vi "测棒价值数据处理.vi"() -> ()   [LabVIEW 2020]
uses:
  <vilib>/Utility/miscctls.llb/LVAnnotationListTypeDef.ctl
  <vilib>/Utility/miscctls.llb/LVRowAndColumnTypeDef.ctl
  <vilib>/Utility/inputDevices.llb/mouseAcquire.vi
  <vilib>/Analysis/NI_AALPro.lvlib
panel:
  out "准临界周期 (s)":dbl[](array[numeric])
  out "拟合反应性 (pcm)":dbl[](array[numeric])
  out "终端反应性 (pcm)":dbl[](array[numeric])
  out "实时反应性 (pcm)":dbl[](array[numeric])
  in  "刻棒选择":u16(ring)
  in  "棒位偏移":dbl(slide) min=-0.1 max=0.1 step=0.001 scale=-0.1..0.1 scale format="%#.3g"
  in  "反应性标尺":bool
  in  "Min+":bool
  in  "Min-":bool
  in  "Max+":bool
  in  "Max-":bool
  out "历史波形图":dbl[][](graph)
  in  "曲线标尺":bool[](array[boolean])=[TRUE, TRUE]
  in  "曲线隐显":bool[](array[boolean])=[TRUE, TRUE, FALSE, FALSE, FALSE]
  out "终端":i32
  out "动态段":i32
  out "左选标时刻":timestamp
  out "总时长":dbl
  in  "开始计算":bool
  in  "重选文件":bool
  in  "退出程序":bool
  out "filepath":path caption="数据文件路径和名称"
  out "数据采集起止时间":string
  out "临界段":i32
  out "稳定临界":i32
  out "开始落棒":i32
  out "Table":string[][](table) caption="总价值汇总"
  in  "保存表格":bool
  in  "添加记录":bool
  in  "选项卡控件":enum32{"动态段数据", "动态段曲线"}(tab)
  out "ValueTable":string[][](table)=[["102.000000", "NaN", "-348.352776", "7.241968"], ["101.000000", "NaN", "2474.422828", "-4.851056"], ["100.000000", "NaN", "-622.831158", "13.483680"], ["99.000000", "NaN", "-527.371545", "-19.758989"], ["98.000000", "NaN", "-567.571450", "-10.039112"], ["97.000000", "NaN", "-587.204400", "6.175295"], ["96.000000", "NaN", "-348.236291", "13.619997"], ["95.000000", "NaN", "2458.347144", "-10.205061"], ["94.000000", "NaN", "-622.921258", "5.615908"], ["93.000000", "NaN", "-527.356225", "2.660273"], ["92.000000", "NaN", "-567.556832", "-0.988388"], ["91.000000", "NaN", "-587.208474", "-1.085916"], ["90.000000", "NaN", "-351.120934", "-4.397986"], ["89.000000", "NaN", "2304.904029", "2.228443"], ["88.000000", "NaN", "-618.140019", "-11.538202"], ["87.000000", "NaN", "-525.138329", "-21.395784"], ["86.000000", "NaN", "-565.982171", "-3.062838"], ["85.000000", "NaN", "-585.993836", "-11.582806"], ["84.000000", "NaN", "-356.379876", "-4.609295"], ["83.000000", "NaN", "2014.719947", "-24.758602"], ["82.000000", "NaN", "-607.663750", "-9.042081"], ["81.000000", "NaN", "-519.521004", "-11.768277"], ["80.000000", "NaN", "-561.868691", "-21.104680"], ["79.000000", "NaN", "-582.802468", "-20.175712"], ["78.000000", "NaN", "-370.631005", "-22.793518"], ["77.000000", "NaN", "1553.766334", "-35.673673"], ["76.000000", "NaN", "-582.848588", "-30.558160"], ["75.000000", "NaN", "-506.097573", "-43.964250"], ["74.000000", "NaN", "-552.008980", "-40.812654"], ["73.000000", "NaN", "-575.099190", "-48.470411"], ["72.000000", "NaN", "-396.508813", "-49.474470"], ["71.000000", "NaN", "1094.646827", "-51.345674"], ["70.000000", "NaN", "-538.590142", "-76.883382"], ["69.000000", "NaN", "-482.233040", "-72.882963"], ["68.000000", "NaN", "-534.351227", "-82.754262"], ["67.000000", "NaN", "-561.206460", "-96.003896"], ["66.000000", "NaN", "-437.894280", "-90.676832"], ["65.000000", "NaN", "754.871925", "-96.218252"], ["64.000000", "NaN", "-475.456872", "-112.709539"], ["63.000000", "NaN", "-448.215874", "-123.690824"], ["62.000000", "NaN", "-508.844033", "-113.615911"], ["61.000000", "NaN", "-540.932023", "-115.695623"], ["60.000000", "NaN", "-505.853066", "-123.674741"], ["59.000000", "NaN", "533.852882", "-168.205152"], ["58.000000", "NaN", "-398.363793", "-171.710203"], ["57.000000", "NaN", "-411.278634", "-156.485715"], ["56.000000", "NaN", "-503.550530", "-189.779630"], ["55.000000", "NaN", "-558.146439", "-200.472120"], ["54.000000", "NaN", "-602.408646", "-192.425687"], ["53.000000", "NaN", "-639.806430", "-193.738553"], ["52.000000", "NaN", "-674.476414", "-191.523603"], ["51.000000", "NaN", "-700.441693", "-249.642133"], ["50.000000", "NaN", "-724.497986", "-241.971433"], ["49.000000", "NaN", "-754.798043", "-266.290555"], ["48.000000", "NaN", "-775.840317", "-264.434385"], ["47.000000", "NaN", "-798.536919", "-291.856107"], ["46.000000", "NaN", "-818.504510", "-287.589536"], ["45.000000", "NaN", "-838.204919", "-305.410093"], ["44.000000", "NaN", "-860.447259", "-298.660703"], ["43.000000", "NaN", "-884.024087", "-330.586606"], ["42.000000", "NaN", "-908.885247", "-345.129301"], ["41.000000", "NaN", "-937.339654", "-354.504972"], ["40.000000", "NaN", "-955.449700", "-356.992582"], ["39.000000", "NaN", "-990.566125", "-360.303831"], ["38.000000", "NaN", "-1010.004540", "-374.933347"], ["37.000000", "NaN", "-1043.396813", "-401.850858"], ["36.000000", "NaN", "-1071.659783", "-439.057493"], ["35.000000", "NaN", "-1099.095025", "-406.192869"], ["34.000000", "NaN", "-1152.078759", "-466.934385"], ["33.000000", "NaN", "-1177.829796", "-468.282712"], ["32.000000", "NaN", "-1222.924279", "-456.289701"], ["31.000000", "NaN", "-1264.624718", "-460.500486"], ["30.000000", "NaN", "-1309.989220", "-475.509641"], ["29.000000", "NaN", "-1367.020409", "-503.021970"], ["28.000000", "NaN", "-1422.772057", "-497.549833"], ["27.000000", "NaN", "-1496.451501", "-486.375333"], ["26.000000", "NaN", "-1576.901635", "-506.166898"], ["25.000000", "NaN", "-1667.238000", "-603.034665"], ["24.000000", "NaN", "-1761.502953", "-538.524656"], ["23.000000", "NaN", "-2206.159569", "-566.865903"], ["22.000000", "NaN", "-1641.630273", "-535.883054"], ["21.000000", "NaN", "-1600.580163", "-573.607480"], ["20.000000", "NaN", "-1556.563500", "-559.440488"], ["19.000000", "NaN", "-1515.641564", "-582.165281"], ["18.000000", "NaN", "-1478.138878", "-558.577390"], ["17.000000", "NaN", "-1443.844872", "-665.358335"], ["16.000000", "NaN", "-1412.422997", "-573.492002"], ["15.000000", "NaN", "-1383.463097", "-615.937436"], ["14.000000", "NaN", "-1356.686242", "-644.269102"], ["13.000000", "NaN", "-634.271134", "-622.237424"], ["12.000000", "NaN", "12773.841041", "-573.894834"], ["11.000000", "NaN", "-2338.911156", "-625.372129"], ["10.000000", "NaN", "-1151.127679", "-629.015623"], ["9.000000", "NaN", "-1188.514062", "-614.873228"], ["8.000000", "NaN", "-1188.497399", "-642.504880"], ["7.000000", "NaN", "-1181.560387", "-654.091062"], ["6.000000", "NaN", "-1171.780419", "-630.052976"], ["5.000000", "NaN", "-1160.657616", "-647.022458"], ["4.000000", "NaN", "-1149.016137", "-624.654294"], ["3.000000", "NaN", "-1136.935021", "-613.506833"], ["2.000000", "NaN", "-1124.845116", "-602.012571"], ["1.000000", "NaN", "-777.317902", "-666.974668"]] caption="动态段"
  in  "另存数据":bool
  out "价值曲线":cluster{dbl[], dbl[]}[](graph) caption="（X和Y数组）多曲线"
  out "提示信息":string
  # "手动"
  # "自动"
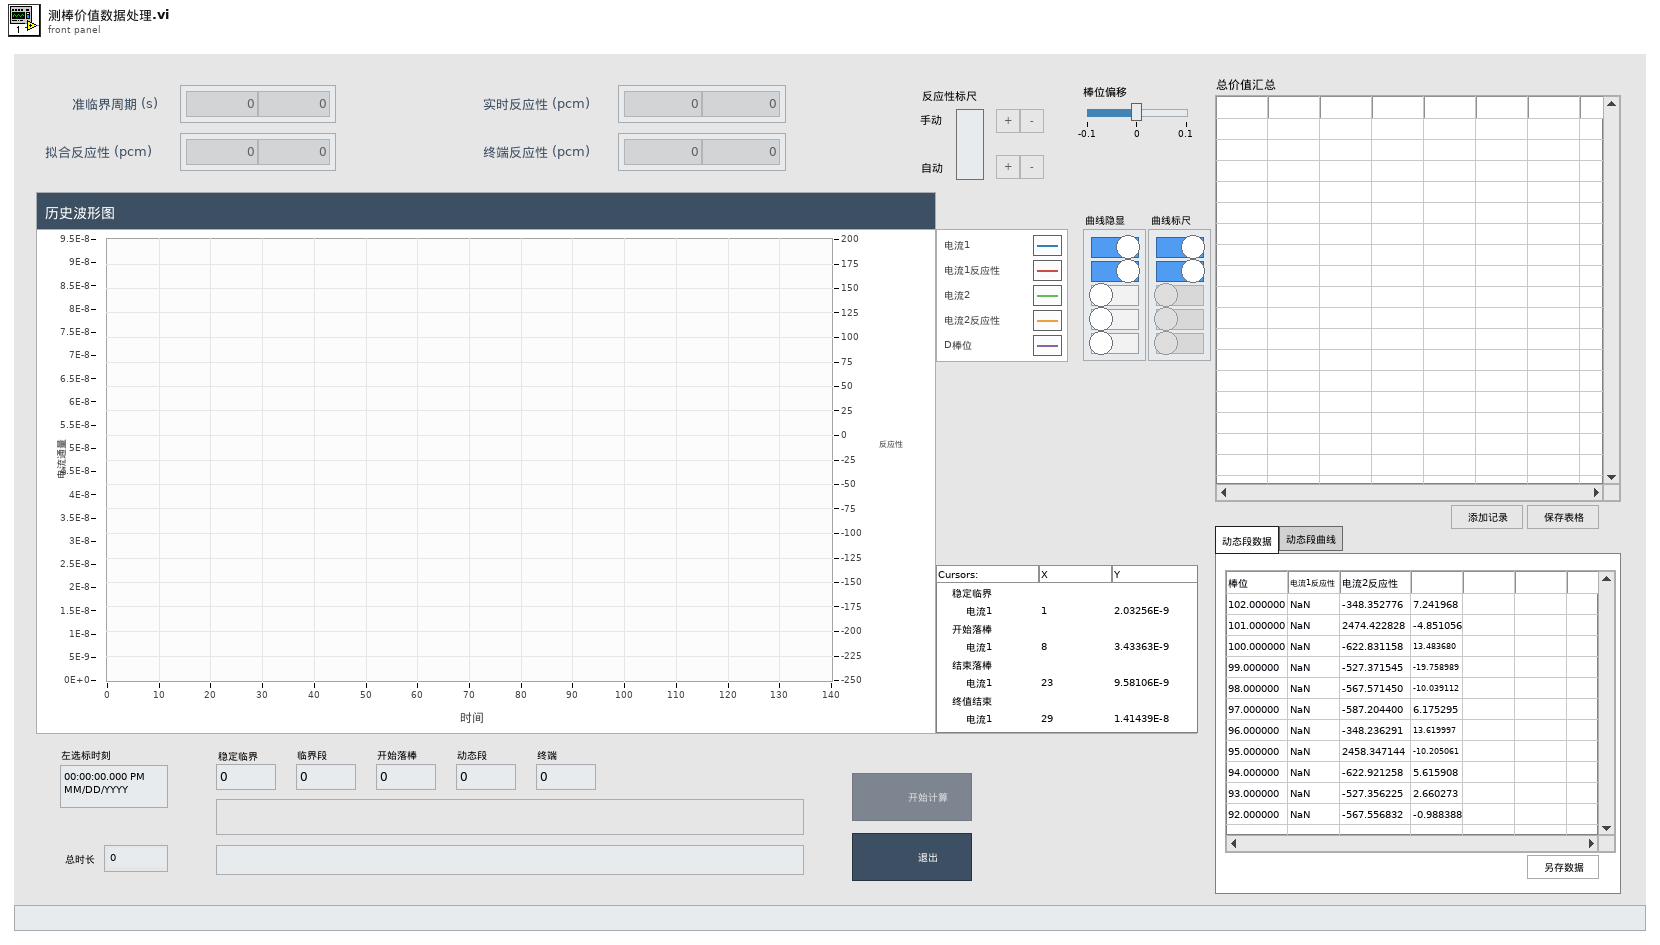
[diagram p1: front panel]
types:
  T1 = enum8{"Enabled", "Disabled", "Disabled and Grayed Out"}
  T2 = typedef "LVAnnotationListTypeDef.ctl" = cluster{"Name":string, "Color":u32, "Style":u8, "Point Style":u8, "Name Visible":bool, "Allow Drag":bool, "Annotation Mode":u32, "Plot":i32, "Index":i32, "Position":cluster{"X":dbl, "Y":dbl}, "X Scale":u32, "Y Scale":u32, "Show Arrow":bool, "Lock Name":bool, "Plot Area":i32, "Label Offset":cluster{"X":dbl, "Y":dbl}}[]
  T3 = cluster{"Name":string, "Color":u32, "Style":u8, "Point Style":u8, "Name Visible":bool, "Allow Drag":bool, "Annotation Mode":u32, "Plot":i32, "Index":i32, "Position":cluster{"X":dbl, "Y":dbl}, "X Scale":u32, "Y Scale":u32, "Show Arrow":bool, "Lock Name":bool, "Plot Area":i32, "Label Offset":cluster{"X":dbl, "Y":dbl}}
  T4 = cluster{"amp min":dbl, "amp max":dbl, "damping min":dbl, "damping max":dbl, "offset min":dbl, "offset max":dbl}
  T5 = enum16{"open", "replace", "create", "open or create", "replace or create", "replace or create with confirmation"}
  T6 = typedef "LVRowAndColumnTypeDef.ctl" = cluster{"Row":i32, "Column":i32}
  T7 = typedef "LVCursorListTypeDef.ctl" = cluster{"Name":string, "Color":u32, "Style":u8, "Point Style":u8, "Name Visible":bool, "Allow Drag":bool, "Cursor Mode":u32, "Plot":i32, "Index":i32, "Position":cluster{"X":dbl, "Y":dbl}, "X Scale":u32, "Y Scale":u32, "Watch Plots":i32[], "Watch All Plots":bool, "Plot Area":i32, "Label Offset":cluster{"X":dbl, "Y":dbl}}[]
  T8 = cluster{"button 1":bool, "button 2":bool, "button 3":bool, "button 4":bool}
  T9 = cluster{"Name":string, "Color":u32, "Style":u8, "Point Style":u8, "Name Visible":bool, "Allow Drag":bool, "Cursor Mode":u32, "Plot":i32, "Index":i32, "Position":cluster{"X":dbl, "Y":dbl}, "X Scale":u32, "Y Scale":u32, "Watch Plots":i32[], "Watch All Plots":bool, "Plot Area":i32, "Label Offset":cluster{"X":dbl, "Y":dbl}}
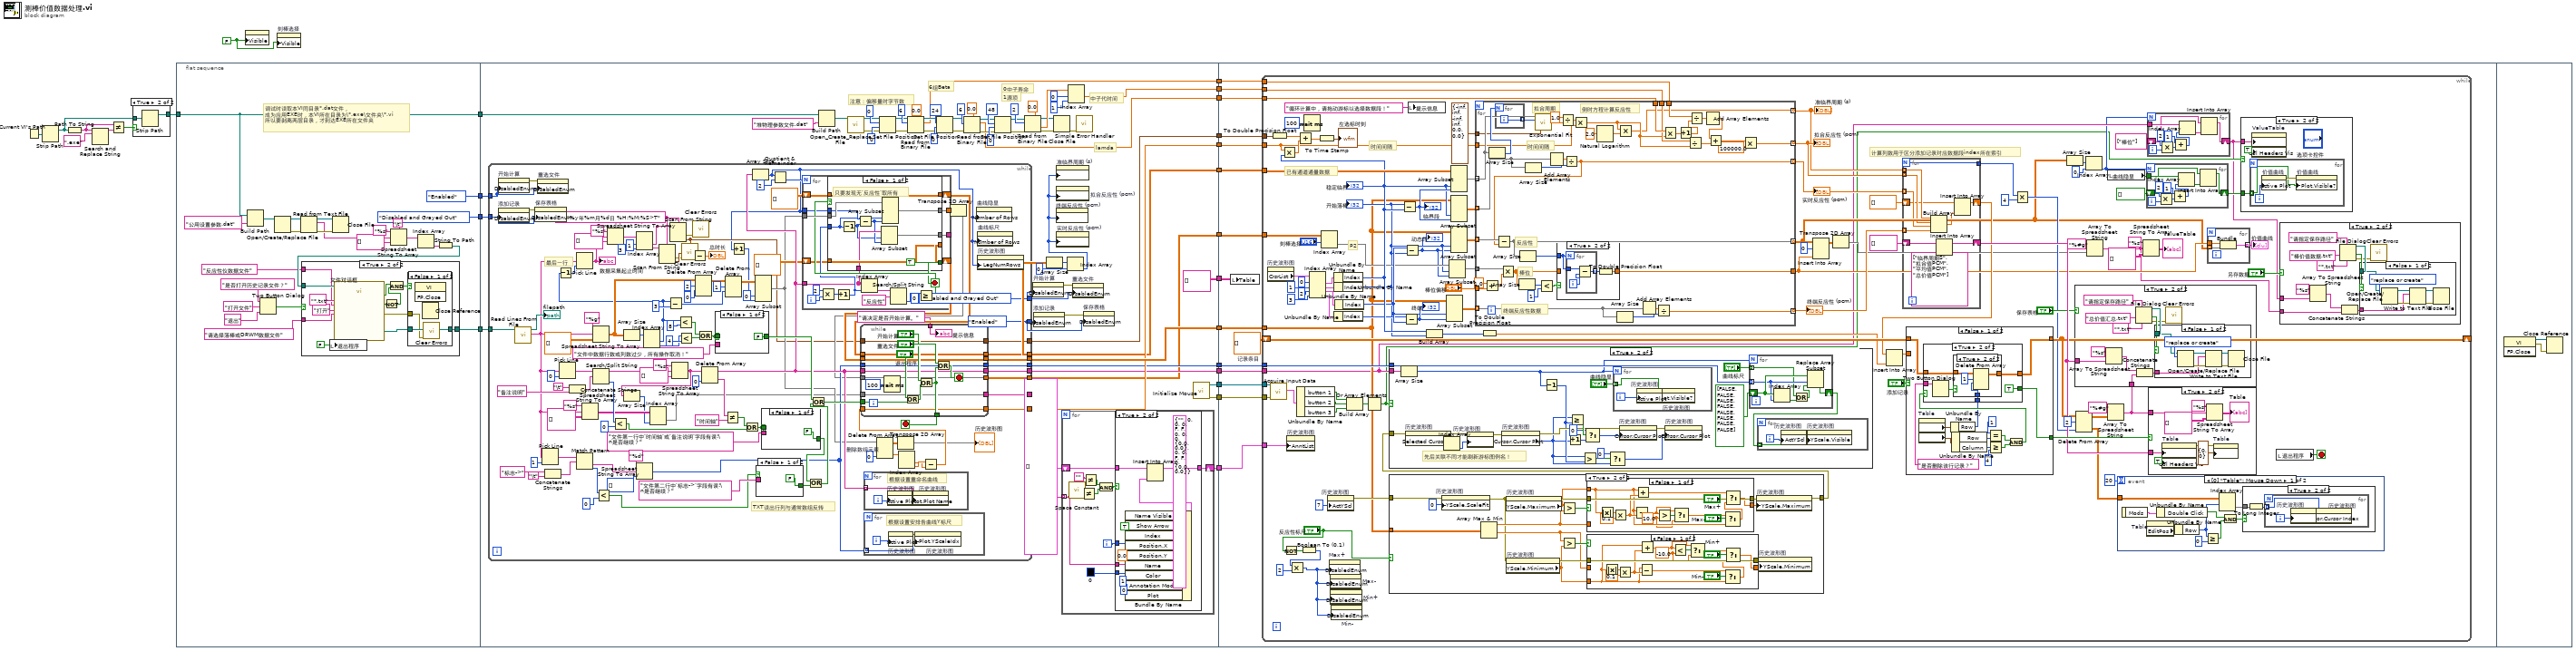
[diagram p0: block diagram]
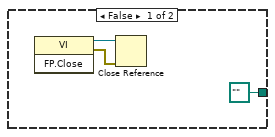
[diagram p3: hidden frame]
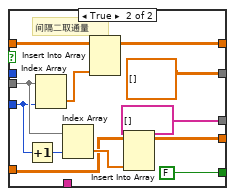
[diagram p6: hidden frame]
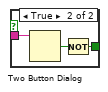
[diagram p7: hidden frame]
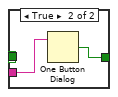
[diagram p8: hidden frame]
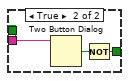
[diagram p9: hidden frame]
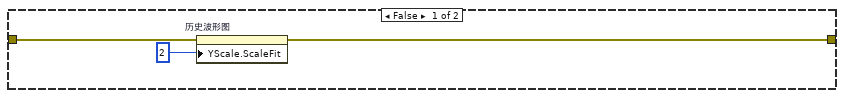
[diagram p13: hidden frame]
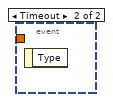
[diagram p17: hidden frame]
diagram:
  w1 = FALSE ("Visible")
  n1 = Current VI's Path() -> (path=w5:path)
  n2 = Strip Path(path=w5) -> (stripped path=w10:path)  [unwired: 1 out]
  n3 = Path To String(path=w10) -> (string=w8:string)
  n4 = Search and Replace String(input string=w8, search string=".exe" ("搜索字符串")) -> (result string=w7:string)  [unwired: 6 in, 3 out]
  n5 = Not Equal?(x=w8, y=w7) -> (x != y?=w9:bool)
  n6 = case shown="True" w9 {
    tunnel: w10 -> [w27 w29]
    tunnel: [w27 w28] -> w3
    frame False {
    }
    frame True {
      n7 = Strip Path(path=w29) -> (stripped path=w28:path)  [unwired: 1 out]
    }
  }
  n8 = flat-sequence {
    tunnel: [T1."Enabled" ("禁用")] -> w14
    tunnel: [T1."Disabled and Grayed Out" ("禁用")] -> w13
    tunnel: [w30] -> w4
    tunnel: w3 -> [w30]
    tunnel: [w31] -> w2
    tunnel: [w97] -> w26
    tunnel: [w96] -> w25
    tunnel: [w95] -> w24
    tunnel: [w100] -> w23
    tunnel: [w99] -> w22
    tunnel: [w98] -> w21
    tunnel: [w91] -> w20
    tunnel: [w90] -> w19
    tunnel: [w89] -> w18
    tunnel: [w88] -> w17
    tunnel: [w86] -> w16
    tunnel: [string[][] [] ("添加的数组")] -> w15
    tunnel: w14 -> [w81]
    tunnel: w13 -> [w78]
    tunnel: [w77] -> w12
    tunnel: [w76] -> w11
    tunnel: w4 -> [w75]
    tunnel: w2 -> [w74]
    tunnel: w24 -> [w359]
    tunnel: w26 -> [w358]
    tunnel: w25 -> [w357]
    tunnel: w23 -> [w356]
    tunnel: w22 -> [w355]
    tunnel: w21 -> [w354]
    tunnel: w20 -> [w353]
    tunnel: w19 -> [w352]
    tunnel: w18 -> [w351]
    tunnel: w17 -> [w350]
    tunnel: w16 -> [w349]
    tunnel: w15 -> [w347]
    tunnel: w12 -> [w346]
    tunnel: w11 -> [w345]
    frame #0 {
      # "调试时读取本VI同目录*.dat文件，\n成为应用EXE时，本VI所在目录为\\*.exe\\文件夹\\*.vi\n所以要剥离两层目录，才到达EXE所在文件夹"
      n9 = Build Path(base path=w30, name or relative path="公用设置参数.dat") -> (appended path=w45:path)
      n10 = Two Button Dialog(message="是否打开历史记录文件？", 1:"退出" ("message"), 2:"打开文件" ("message")) -> (T button?=w35:bool)
      n11 = Open/Create/Replace File(file path (use dialog)=w45) -> (refnum out=w42:refnum<file>, error out=w41:errorcluster)  [unwired: 5 in, 1 out]
      n12 = Read from Text File(file (use dialog)=w42, error in=w41) -> (refnum out=w43:refnum<file>, text=w37:string, error out=w44:errorcluster)  [unwired: 1 in, 2 out]
      n13 = Close File(refnum=w43, error in=w44) -> ()  [unwired: 2 out]
      n14 = Spreadsheet String To Array(delimiter (Tab)="\t", format string="%s", spreadsheet string=w37, array type (2D Dbl)=string[] [] ("添加的数组")) -> (array=w36:string[])
      n15 = Index Array(array=w36) -> (element=w47:string)  [unwired: 1 in]
      n16 = String To Path(string=w47) -> (path=w34:path)
      n17 = case shown="True" w35 {
        tunnel: w34 -> [_ w68]
        tunnel: "请选择落棒或DRWM数据文件" ("prompt") -> [_ w64]
        tunnel: "反应性仪数据文件" ("pattern label") -> [_ w63]
        tunnel: [path "" ("selected path") w61] -> w31
        frame False {
          n18 = invoke class="VI" method="FP.Close"() -> (reference out=w53:refnum<vi>, error out=w54:errorcluster)  [unwired: 3 in, 1 out]
          n19 = Close Reference(reference=w53, error in (no error)=w54) -> ()  [unwired: 1 out]
        }
        frame True {
          n20 = local write "退出程序"(FALSE ("退出程序")) -> ()
          n21 = call "文件对话框"("start path"=w68, "prompt"=w64, "button label"="打开", "pattern (all files)"="*.txt", "pattern label"=w63) -> ("selected path"=w62:path, "exists"=w59:bool, "cancelled"=w60:bool, "error out"=w56:errorcluster)  [unwired: 7 in]
          n22 = Not(x=w60) -> (.not. x?=w58:bool)
          n23 = And(x=w59, y=w58) -> (x .and. y?=w57:bool)
          n24 = case shown="False" w57 {
            tunnel: w62 -> [w72 w73]
            tunnel: [w72 w73] -> w61
            tunnel: w56 -> [w69 _]
            frame False {
              n25 = invoke class="VI" method="FP.Close"() -> (reference out=w70:refnum<vi>, error out=w71:errorcluster)  [unwired: 3 in, 1 out]
              n26 = Close Reference(reference=w70, error in (no error)=w71) -> ()  [unwired: 1 out]
              n27 = call <vilib>:"Clear Errors.vi"("error in (no error)"=w69) -> ()  [unwired: 5 in, 2 out]
            }
            frame True {
            }
          }
        }
      }
    }
    frame #1 {
      # "注意：偏移量时字节数"
      # "0中子寿命"
      # "1源项"
      # "6组Beta"
      # "中子代时间"
      # "lamda"
      n28 = while {
        tunnel: [w213] -> w97
        tunnel: [w261] -> w91
        tunnel: [w210] -> w90
        tunnel: [w211] -> w95
        tunnel: [w199] -> w96
        tunnel: [w184] -> w87
        tunnel: [T1."Disabled and Grayed Out" ("禁用")] -> w82
        tunnel: w81 -> [w180]
        tunnel: [T1."Enabled" ("禁用")] -> w79
        tunnel: w78 -> [w177]
        tunnel: [w173] -> w77
        tunnel: [w158] -> w76
        tunnel: w74 -> [w157]
        stop <- w267 stop-if-true
        w164 = "%<%y年%m月%d日 %H:%M:%S>T" ("格式字符串")
        # "TXT读出行列与通常数组反转"
        # "最后一行"
        n29 = property on="开始计算" class="Bool"("DisabledEnum"=w180) -> (error out=w181:errorcluster)  [unwired: 2 in, 1 out]
        n30 = property on="添加记录" class="Bool"("DisabledEnum"=w177) -> (error out=w178:errorcluster)  [unwired: 2 in, 1 out]
        n31 = call <vilib>:"Read Lines From File.vi"("file path (dialog if empty)"=w157) -> ("new file path (Not A Path if cancelled)"=→"filepath":path, "line string"=w189:string)  [unwired: 5 in, 2 out]
        n32 = property on="保存表格" class="Bool"(error in=w178, "DisabledEnum"=w177) -> ()  [unwired: 1 in, 2 out]
        n33 = property on="重选文件" class="Bool"(error in=w181, "DisabledEnum"=w180) -> ()  [unwired: 1 in, 2 out]
        n34 = Pick Line(multi-line string=w189, line index=1 ("行索引")) -> (output string=w240:string)  [unwired: 1 in]
        n35 = Concatenate Strings("标志->" ("搜索字符串/字符(-)"), "\t") -> (w237:string)
        n36 = Pick Line(multi-line string=w189, line index=0 ("行索引")) -> (output string=w259:string)  [unwired: 1 in]
        n37 = Concatenate Strings("\t", "备注说明" ("搜索字符串/字符(-)")) -> (w220:string)
        n38 = Match Pattern(string=w240, regular expression=w237) -> (after substring=w234:string, offset past match=w228:i32)  [unwired: 1 in, 2 out]
        n39 = Spreadsheet String To Array ("电子表格字符串至数组转换")(format string="%s" ("format (%.3f)"), spreadsheet string=w189, array type (2D Dbl)=string[][] [] ("添加的数组")) -> (array=w188:string[][])  [unwired: 1 in]
        n40 = Spreadsheet String To Array ("电子表格字符串至数组转换")(format string="%g" ("format (%.3f)"), spreadsheet string=w189, array type (2D Dbl)=dbl[][] [] ("type (empty)")) -> (array=w222:dbl[][])  [unwired: 1 in]
        n41 = Search/Split String(string=w259, search string/char (-)=w220) -> (substring before match=w258:string, offset of match=w257:i32)  [unwired: 1 in, 1 out]
        n42 = Less?(x=w228, y=0) -> (x < y?=w227:bool)
        n43 = Less?(x=w257, y=0) -> (x < y?=w254:bool)
        n44 = Array Size(array=w222) -> (size(s)=w268:i32[])
        n45 = Spreadsheet String To Array ("电子表格字符串至数组转换")(format string="%d" ("format (%.3f)"), spreadsheet string=w234, array type (2D Dbl)=i32[] [] ("添加的数组")) -> (array=w208:i32[])  [unwired: 1 in]
        n46 = Index Array(array=w268) -> (element #1=w174:i32, element #2=w248:i32)  [unwired: 2 in]
        n47 = Decrement(x=w174) -> (x-1=w175:i32)
        n48 = Pick Line(multi-line string=w189, line index=w175) -> (output string=w172:string)  [unwired: 1 in]
        "数据采集起止时间" <- w172
        n49 = Spreadsheet String To Array(format string="%s" ("格式字符串"), spreadsheet string=w172, array type (2D Dbl)=string[] [] ("添加的数组")) -> (array=w169:string[])  [unwired: 1 in]
        n50 = Index Array(array=w169, index #1=1 ("索引"), index #2=3 ("索引")) -> (element #1=w166:string, element #2=w165:string)
        n51 = Scan From String(format string=w164, input string=w165) -> (error out=w159:errorcluster, output 1=w163:timestamp)  [unwired: 3 in, 2 out]
        n52 = Subtract(x=w174, y=3) -> (x-y=w217:i32)
        n53 = Scan From String(format string=w164, input string=w166) -> (error out=w160:errorcluster, output 1=w162:timestamp)  [unwired: 3 in, 2 out]
        n54 = Spreadsheet String To Array ("电子表格字符串至数组转换")(format string="%s" ("format (%.3f)"), spreadsheet string=w258, array type (2D Dbl)=string[] [] ("添加的数组")) -> (array=w187:string[])  [unwired: 1 in]
        n55 = Array Size(array=w187) -> (size(s)=w186:i32)
        n56 = Index Array(array=w188, index (col)=w186) -> (element=w185:string[])  [unwired: 1 in]
        n57 = Less?(x=w174, y=8) -> (x < y?=w246:bool)
        n58 = Less?(x=w248, y=4) -> (x < y?=w245:bool)
        n59 = call <vilib>:"Clear Errors.vi"("error in (no error)"=w159) -> ()  [unwired: 5 in, 2 out]
        n60 = Subtract(x=w163, y=w162) -> (x-y=→"总时长":dbl)
        n61 = call <vilib>:"Clear Errors.vi"("error in (no error)"=w160) -> ()  [unwired: 5 in, 2 out]
        n62 = Delete From Array(array=w222, length=2 ("长度"), index (row)=0 ("索引")) -> (array with subset deleted=w221:dbl[][])  [unwired: 1 in, 1 out]
        n63 = Or(x=w246, y=w245) -> (x .or. y?=w247:bool)
        n64 = Delete From Array(array=w187, index=0 ("索引")) -> (deleted portion=w196:string, array with subset deleted=w209:string[])  [unwired: 1 in]
        n65 = case shown="False" w247 {
          tunnel: w247 -> [_ _]
          tunnel: [FALSE w322] -> w242
          tunnel: "文件中数据行数或列数过少，所有操作取消！" ("y") -> [_ w323]
          frame False {
          }
          frame True {
            n66 = One Button Dialog(message=w323) -> (true=w322:bool)  [unwired: 1 in]
          }
        }
        n67 = Not Equal?(x=w196, y="时间轴") -> (x != y?=w253:bool)
        n68 = Delete From Array(array=w221, length=1 ("长度"), index (row)=w217) -> (array with subset deleted=w195:dbl[][])  [unwired: 1 in, 1 out]
        n69 = Or(x=w253, y=w254) -> (x .or. y?=w252:bool)
        n70 = Array Size(array=w209) -> (size(s)=w155:i32)
        n71 = Increment(x=w155) -> (x+1=w192:i32)
        n72 = Array Subset(array=w195, index (col)=0 ("索引"), length (col)=w192) -> (w194:dbl[][])  [unwired: 2 in]
        n73 = case shown="False" w227 {
          tunnel: "文件第二行中‘标志->’字段有误!\n是否继续？" ("y") -> [_ w320]
          tunnel: [FALSE w318] -> w232
          frame False {
          }
          frame True {
            n74 = Two Button Dialog(message=w320) -> (T button?=w319:bool)  [unwired: 2 in]
            n75 = Not(x=w319) -> (.not. x?=w318:bool)
          }
        }
        n76 = case shown="False" w252 {
          tunnel: w252 -> [_ _]
          tunnel: "文件第一行中‘时间轴’或‘备注说明’字段有误!\n是否继续？" ("y") -> [_ w327]
          tunnel: [FALSE w325] -> w231
          frame False {
          }
          frame True {
            n77 = Two Button Dialog(message=w327) -> (T button?=w326:bool)  [unwired: 2 in]
            n78 = Not(x=w326) -> (.not. x?=w325:bool)
          }
        }
        n79 = Quotient & Remainder(x=w155, y=2) -> (floor(x/y)=w214:i32)  [unwired: 1 out]
        n80 = for {
          N: w214 -> [_]
          tunnel: w194 -> [w287]
          tunnel: w209 -> [w276]
          shift-right: [w285] -> w198
          shift-left: dbl[][] [] ("type (empty)") -> [w286]
          tunnel: w155 -> [w281]
          tunnel: [w280] -> w212
          shift-right: [w277] -> w204
          shift-left: dbl[][] [] ("type (empty)") -> [w278]
          tunnel: [w275] -> _
          i -> [w293]
          stop <- w282 stop-if-true
          n81 = Multiply(x=2, y=w293) -> (x*y=w279:i32)
          n82 = Increment(x=w279) -> (x+1=w283:i32)
          n83 = Index Array(array=w276, index=w283) -> (element=w291:string)
          n84 = Search/Split String(string=w291, search string/char (-)="反应性" ("搜索字符串/字符(-)")) -> (offset of match=w289:i32)  [unwired: 1 in, 2 out]
          n85 = Greater Or Equal?(x=w289, y=0) -> (x >= y?=w284:bool)
          n86 = case shown="False" w284 {
            tunnel: w287 -> [w302 w311]
            tunnel: w286 -> [w304 w316]
            tunnel: [w304 w314] -> w285
            tunnel: w283 -> [w297 w306]
            tunnel: [TRUE FALSE] -> w282
            tunnel: w281 -> [w301 _]
            tunnel: [w300 dbl[][] [] ("type (empty)")] -> w280
            tunnel: w278 -> [w299 w309]
            tunnel: [w299 w308] -> w277
            tunnel: w276 -> [w298 _]
            tunnel: [w295 string[] []] -> w275
            frame False {
              # "只要发现无‘反应性’取所有"
              n87 = Decrement(x=w297) -> (x-1=w294:i32)
              n88 = Subtract(x=w301, y=w294) -> (x-y=w296:i32)
              n89 = Array Subset(array=w298, index=w294, length=w296) -> (w295:string[])
              n90 = Array Subset(array=w302, index (col)=w297, length (col)=w296) -> (w300:dbl[][])  [unwired: 2 in]
            }
            frame True {
              # "间隔二取通量"
              n91 = Increment(x=w306) -> (x+1=w307:i32)
              n92 = Index Array(array=w311, index (col)=w306) -> (element=w315:dbl[])  [unwired: 1 in]
              n93 = Index Array(array=w311, index (col)=w307) -> (element=w310:dbl[])  [unwired: 1 in]
              n94 = Insert Into Array(array=w316, new element=w315) -> (w314:dbl[][])  [unwired: 2 in]
              n95 = Insert Into Array(array=w309, new element=w310) -> (w308:dbl[][])  [unwired: 2 in]
            }
          }
        }
        n96 = Or(x=w231, y=w232) -> (x .or. y?=w230:bool)
        n97 = Or(x=w242, y=w230) -> (x .or. y?=w243:bool)
        n98 = for {
          tunnel: w209 -> [w273] mode=indexing
          i -> [w274]
          # "根据设置重命名曲线"
          n99 = property on="历史波形图" class="WFGraph (strict)"("Active Plot"=w274) -> (error out=w272:errorcluster)  [unwired: 2 in, 1 out]
          n100 = property on="历史波形图" class="WFGraph (strict)"(error in=w272, "Plot.Plot Name"=w273) -> ()  [unwired: 1 in, 2 out]
        }
        n101 = for {
          tunnel: w208 -> [w269] mode=indexing
          i -> [w271]
          # "根据设置安排各曲线Y标尺"
          n102 = property on="历史波形图" class="WFGraph (strict)"("Active Plot"=w271) -> (error out=w270:errorcluster)  [unwired: 2 in, 1 out]
          n103 = property on="历史波形图" class="WFGraph (strict)"(error in=w270, "Plot.YScaleIdx"=w269) -> ()  [unwired: 1 in, 2 out]
        }
        n104 = Delete From Array "删除数组元素"(array=w194, index (col)=0 ("禁用的索引 (列)")) -> (deleted portion=w203:dbl[], array with subset deleted=w207:dbl[][])  [unwired: 2 in]
        n105 = Transpose 2D Array(2D array=w207) -> (transposed array=→"历史波形图":dbl[][])
        n106 = Index Array(array=w203) -> (element #1=w201:dbl, element #2=w202:dbl)  [unwired: 2 in]
        n107 = Subtract(x=w202, y=w201) -> (x-y=w200:dbl)
        n108 = Transpose 2D Array(2D array=w212) -> (transposed array=w183:dbl[][])
        n109 = while {
          tunnel: [w335] -> w213
          tunnel: [w333] -> w261
          tunnel: w204 -> [w335]
          tunnel: w209 -> [w333]
          tunnel: [w342] -> w267
          tunnel: w243 -> [w338]
          tunnel: w198 -> [w336]
          tunnel: [w336] -> w211
          tunnel: w208 -> [w334]
          tunnel: [w334] -> w210
          tunnel: w200 -> [w332]
          tunnel: [w332] -> w199
          tunnel: "请决定是否开始计算。" ("提示信息") -> [w331]
          tunnel: [w330] -> w184
          tunnel: w185 -> [w330]
          tunnel: [w329] -> w158
          tunnel: w183 -> [w329]
          tunnel: [w328] -> w173
          tunnel: w162 -> [w328]
          stop <- w341 stop-if-true
          n110 = Wait (ms)(milliseconds to wait=u32 100 ("等待时间（毫秒）")) -> ()  [unwired: 1 out]
          n111 = Or(x="退出程序", y=w338) -> (x .or. y?=w339:bool)
          n112 = Or(x="开始计算", y=w339) -> (x .or. y?=w342:bool)
          n113 = Or(x="重选文件", y=w342) -> (x .or. y?=w341:bool)
          "提示信息" <- w331
        }
        n114 = property on="曲线隐显" class="Arr (strict)"("Number of Rows"=w155) -> ()  [unwired: 2 in, 2 out]
        n115 = property on="曲线标尺" class="Arr (strict)"("Number of Rows"=w155) -> ()  [unwired: 2 in, 2 out]
        n116 = property on="历史波形图" class="WFGraph (strict)"("LegNumRows"=w155) -> ()  [unwired: 2 in, 2 out]
      }
      n117 = Build Path(base path=w75, name or relative path="堆物理参数文件.dat" ("string")) -> (appended path=w116:path)
      n118 = call <vilib>:"Open_Create_Replace File.vi"("file path"=w116) -> ("error out"=w101:errorcluster, "refnum"=w102:refnum<file>)  [unwired: 7 in, 2 out]
      n119 = Set File Position(offset (in bytes) (0)=0, refnum=w102, from (0:start)=0, error in=w101) -> (refnum out=w113:refnum<file>, error out=w112:errorcluster)
      n120 = Read from Binary File(5:sgl 0.0, 8:w112, 10:6, 11:w113) -> (0:w108:errorcluster, 2:w100:sgl[], 3:w109:refnum<file>)  [unwired: 2 in, 1 out]
      n121 = Set File Position(offset (in bytes) (0)=24, refnum=w109, from (0:start)=0, error in=w108) -> (refnum out=w111:refnum<file>, error out=w110:errorcluster)
      n122 = Read from Binary File(5:sgl 0.0, 8:w110, 10:6, 11:w111) -> (0:w106:errorcluster, 2:w99:sgl[], 3:w107:refnum<file>)  [unwired: 2 in, 1 out]
      n123 = Set File Position(offset (in bytes) (0)=48, refnum=w107, from (0:start)=0, error in=w106) -> (refnum out=w115:refnum<file>, error out=w114:errorcluster)
      n124 = Read from Binary File(5:sgl 0.0, 8:w114, 10:2, 11:w115) -> (0:w104:errorcluster, 2:w124:sgl[], 3:w105:refnum<file>)  [unwired: 2 in, 1 out]
      n125 = property on="开始计算" class="Bool"("DisabledEnum"=w82) -> (error out=w83:errorcluster)  [unwired: 2 in, 1 out]
      n126 = property on="添加记录" class="Bool"("DisabledEnum"=w79) -> (error out=w80:errorcluster)  [unwired: 2 in, 1 out]
      n127 = Array Size(array=w95) -> (size(s)=w94:i32[])
      n128 = Close File(refnum=w105, error in=w104) -> (error out=w103:errorcluster)  [unwired: 1 out]
      n129 = for {
        tunnel: w87 -> [w137] mode=indexing
        shift-right: [w139] -> w86
        shift-left: T2 [] ("注释列表") -> [w140]
        i -> [w141]
        n130 = call <vilib>:"Space Constant.vi"() -> ("String"=w142:string)
        n131 = Not Equal?(x=w142, y=w137) -> (x != y?=w135:bool)
        n132 = Not Equal?(x="", y=w137) -> (x != y?=w136:bool)
        n133 = And(x=w136, y=w135) -> (x .and. y?=w134:bool)
        n134 = case shown="True" w134 {
          tunnel: w137 -> [_ w149]
          tunnel: w141 -> [_ w151]
          tunnel: w140 -> [w143 w154]
          tunnel: [w143 w153] -> w139
          tunnel: u32 0 -> [_ w146]
          frame False {
          }
          frame True {
            w152 = TRUE ("Show Arrow")
            n135 = Bundle By Name(cluster=T3 {"Name"="", "Color"=0, "Style"=0, "Point Style"=0, "Name Visible"=FALSE, "Allow Drag"=FALSE, "Annotation Mode"=0, "Plot"=0, "Index"=0, "Position"={"X"=0.0, "Y"=0.0}, "X Scale"=0, "Y Scale"=0, "Show Arrow"=FALSE, "Lock Name"=FALSE, "Plot Area"=0, "Label Offset"={"X"=0.0, "Y"=0.0}} ("元素"), "Name Visible"=w152, "Show Arrow"=w152, "Index"=w151, "Position.X"=w151, "Position.Y"=0.0 ("Y"), "Name"=w149, "Color"=w146, "Annotation Mode"=u32 1, "Plot"=0) -> (w150:T3)
            n136 = Insert Into Array(array=w154, new element=w150) -> (w153:T2)  [unwired: 1 in]
          }
        }
      }
      n137 = Index Array(array=w94, index=0 ("索引")) -> (element=w93:i32)
      n138 = property on="终端反应性 (pcm)" class="Arr (strict)"("Number of Columns"=w93) -> ()  [unwired: 2 in, 2 out]
      n139 = property on="准临界周期 (s)" class="Arr (strict)"("Number of Columns"=w93) -> ()  [unwired: 2 in, 2 out]
      n140 = property on="拟合反应性 (pcm)" class="Arr (strict)"("Number of Columns"=w93) -> ()  [unwired: 2 in, 2 out]
      n141 = property on="实时反应性 (pcm)" class="Arr (strict)"("Number of Columns"=w93) -> ()  [unwired: 2 in, 2 out]
      n142 = Index Array(array=w124, index #1=0, index #2=1) -> (element #1=w98:sgl)  [unwired: 1 out]
      n143 = property on="重选文件" class="Bool"(error in=w83, "DisabledEnum"=w82) -> ()  [unwired: 1 in, 2 out]
      n144 = call <vilib>:"Simple Error Handler.vi"("error in (no error)"=w103) -> ()  [unwired: 4 in, 5 out]
      n145 = property on="保存表格" class="Bool"(error in=w80, "DisabledEnum"=w79) -> ()  [unwired: 1 in, 2 out]
      n146 = call <vilib>:"Initialize Mouse.vi"() -> ("error out"=w88:errorcluster, "device ID"=w89:refnum<k1>)  [unwired: 1 in, 9 out]
    }
    frame #2 {
      w348 = dbl[][] []  # 记录条目
      n147 = local write "Table"(w347) -> ()
      n148 = while {
        tunnel: w359 -> [w458]
        tunnel: w358 -> [w381]
        tunnel: w357 -> [w408]
        tunnel: w356 -> [w456]
        tunnel: w355 -> [w455]
        tunnel: w354 -> [w454]
        tunnel: w353 -> [w376]
        tunnel: w352 -> [w448]
        tunnel: w351 -> [w446]
        tunnel: w350 -> [w445]
        tunnel: w349 -> [w440]
        shift-right: [w424] -> _
        shift-left: w348 -> [w434]
        tunnel: w346 -> [w413]
        tunnel: w345 -> [w387]
        stop <- w450 stop-if-true
        # "P2"
        # "时间间隔"
        # "计算列数用于区分添加记录对应数据段index所在索引"
        # "已有通道通量数据"
        n149 = property on="历史波形图" class="WFGraph (strict)"() -> ("CrsrList"=w459:T7)  [unwired: 2 in, 2 out]
        n150 = call-poly <vilib>:"Acquire Input Data.vi"("device ID"=w446, "error in (no error)"=w445) -> ("button info"=w447:T8)  [unwired: 1 in, 16 out]
        n151 = To Double Precision Float(number=w413) -> (double precision float=w412:dbl)
        n152 = Not(x="反应性标尺") -> (.not. x?=w364:bool)
        n153 = property on="历史波形图" class="WFGraph (strict)"("AnntList"=w440) -> ()  [unwired: 2 in, 2 out]
        n154 = Unbundle By Name(w447) -> ("button 1"=w444:bool, "button 2"=w443:bool, "button 3"=w442:bool)
        n155 = Boolean To (0,1)(Boolean=w364) -> (0, 1=w362:i16)
        n156 = Multiply(x=w362, y=2) -> (x*y=w360:i32)
        n157 = Wait (ms)(milliseconds to wait=u32 100 ("等待时间（毫秒）")) -> ()  [unwired: 1 out]
        n158 = Index Array(array=w459, index #1=0 ("index"), index #2=1 ("index"), index #3=2 ("索引"), index #4=3 ("索引")) -> (element #1=w461:T9, element #2=w463:T9, element #3=w400:T9, element #4=w399:T9)
        n159 = Index Array(array=w387, index (row)="刻棒选择") -> (element=w386:dbl[])  [unwired: 1 in]
        n160 = property on="历史波形图" class="WFGraph (strict)"("ActYScl"=7 ("活动Y标尺")) -> (error out=w406:errorcluster)  [unwired: 2 in, 1 out]
        n161 = property on="Max+" class="Bool"("DisabledEnum"=w360) -> ()  [unwired: 2 in, 2 out]
        n162 = property on="Max-" class="Bool"("DisabledEnum"=w360) -> ()  [unwired: 2 in, 2 out]
        n163 = property on="Min+" class="Bool"("DisabledEnum"=w360) -> ()  [unwired: 2 in, 2 out]
        n164 = property on="Min-" class="Bool"("DisabledEnum"=w360) -> ()  [unwired: 2 in, 2 out]
        n165 = Unbundle By Name(w461) -> ("Index"=w401:i32)
        "稳定临界" <- w401
        n166 = Multiply(x=w408, y=w401) -> (x*y=w409:dbl)
        n167 = Add(x=w412, y=w409) -> (x+y=w411:dbl)
        n168 = To Time Stamp(1:w411) -> (0:→"左选标时刻":timestamp)
        n169 = Unbundle By Name(w463) -> ("Index"=w385:i32)
        "开始落棒" <- w385
        n170 = Unbundle By Name(w399) -> ("Index"=w396:i32)
        n171 = Unbundle By Name(w400) -> ("Index"=w397:i32)
        n172 = Build Array(w444, w443, w442) -> (w441:bool[])
        n173 = Or Array Elements(Boolean array=w441) -> (logical OR=w368:bool)
        n174 = case shown="True" "反应性标尺" {
          tunnel: w381 -> [_ w522]
          tunnel: w406 -> [w510 w513]
          tunnel: [w509 w512] -> w405
          frame False {
            n175 = property on="历史波形图" class="WFGraph (strict)"(error in=w510, "YScale.ScaleFit"=u8 2 ("Y标尺.标尺调节")) -> (error out=w509:errorcluster)  [unwired: 1 in, 1 out]
          }
          frame True {
            n176 = property on="历史波形图" class="WFGraph (strict)"(error in=w513, "YScale.ScaleFit"=u8 0 ("Y标尺.标尺调节")) -> (error out=w515:errorcluster)  [unwired: 1 in, 1 out]
            n177 = Array Max & Min(array=w522) -> (max value=w524:dbl, min value=w525:dbl)  [unwired: 2 out]
            n178 = property on="历史波形图" class="WFGraph (strict)"(error in=w515) -> (error out=w528:errorcluster, "YScale.Maximum"=w517:dbl)  [unwired: 1 in, 1 out]
            n179 = property on="历史波形图" class="WFGraph (strict)"(error in=w515) -> (error out=w527:errorcluster, "YScale.Minimum"=w516:dbl)  [unwired: 1 in, 1 out]
            n180 = Greater?(x=w517, y=w524) -> (0:w523:bool)
            n181 = Greater?(x=w525, y=w516) -> (0:w526:bool)
            n182 = case shown="False" w523 {
              tunnel: w524 -> [_ w544]
              tunnel: w528 -> [w542 w543]
              tunnel: [w534 w544] -> w521
              tunnel: [w542 w543] -> w520
              tunnel: w517 -> [w533 _]
              frame False {
                w530 = 10.0 ("y")
                n183 = Absolute Value(x=w533) -> (abs(x)=w538:dbl)
                n184 = Multiply(x=w538, y=0.1) -> (x*y=w540:dbl)
                n185 = Subtract(x=w533, y=w540) -> (x-y=w531:dbl)
                n186 = Add(x=w533, y=w540) -> (x+y=w541:dbl)
                n187 = Greater?(x=w531, y=w530) -> (0:w532:bool)
                n188 = Select(t=w531, s=w532, f=w530) -> (s? t:f=w529:dbl)
                n189 = Select(t=w529, s="Max-", f=w533) -> (s? t:f=w535:dbl)
                n190 = Select(t=w541, s="Max+", f=w535) -> (s? t:f=w534:dbl)
              }
              frame True {
              }
            }
            n191 = case shown="False" w526 {
              tunnel: w525 -> [_ w560]
              tunnel: w527 -> [w558 w559]
              tunnel: [w554 w560] -> w519
              tunnel: [w558 w559] -> w518
              tunnel: w516 -> [w550 _]
              frame False {
                w548 = -10.0 ("y")
                n192 = Absolute Value(x=w550) -> (abs(x)=w553:dbl)
                n193 = Multiply(x=w553, y=0.1) -> (x*y=w551:dbl)
                n194 = Subtract(x=w550, y=w551) -> (x-y=w549:dbl)
                n195 = Add(x=w550, y=w551) -> (x+y=w545:dbl)
                n196 = Less?(x=w545, y=w548) -> (x < y?=w547:bool)
                n197 = Select(t=w545, s=w547, f=w548) -> (s? t:f=w546:dbl)
                n198 = Select(t=w549, s="Min-", f=w550) -> (s? t:f=w555:dbl)
                n199 = Select(t=w546, s="Min+", f=w555) -> (s? t:f=w554:dbl)
              }
              frame True {
              }
            }
            n200 = property on="历史波形图" class="WFGraph (strict)"(error in=w520, "YScale.Maximum"=w521) -> (error out=w512:errorcluster)  [unwired: 1 in, 1 out]
            n201 = property on="历史波形图" class="WFGraph (strict)"(error in=w518, "YScale.Minimum"=w519) -> ()  [unwired: 1 in, 2 out]
          }
        }
        n202 = case shown="True" w368 {
          tunnel: w376 -> [_ w643]
          tunnel: w448 -> [_ w657]
          tunnel: w405 -> [_ w644]
          frame False {
          }
          frame True {
            # "先后关联不同才能刷新游标图例名！"
            n203 = Array Size(array=w643) -> (size(s)=w653:i32)
            n204 = property on="历史波形图" class="WFGraph (strict)"(error in=w644) -> (error out=w663:errorcluster, "Selected Cursors"=w665:u32[])  [unwired: 1 in, 1 out]
            n205 = Index Array(array=w665) -> (element=w664:u32)  [unwired: 1 in]
            n206 = property on="历史波形图" class="WFGraph (strict)"(error in=w663, "Active Cursor"=w664) -> (error out=w662:errorcluster)  [unwired: 1 in, 1 out]
            n207 = property on="历史波形图" class="WFGraph (strict)"(error in=w662) -> (error out=w659:errorcluster, "Cursor.Cursor Plot"=w646:i32)  [unwired: 1 in, 1 out]
            n208 = Decrement(x=w653) -> (x-1=w648:i32)
            n209 = Increment(x=w646) -> (x+1=w650:i32)
            n210 = Greater Or Equal?(x=w646, y=w648) -> (x >= y?=w661:bool)
            n211 = Greater?(x=w646, y=w648) -> (0:w649:bool)
            n212 = Select(t=0, s=w661, f=w650) -> (s? t:f=w652:i32)
            n213 = Select(t=0, s=w649, f=w646) -> (s? t:f=w647:i32)
            n214 = for {
              N: w653 -> [_]
              tunnel: "曲线隐显" -> [w669] mode=indexing
              i -> [w670]
              n215 = property on="历史波形图" class="WFGraph (strict)"("Active Plot"=w670) -> (error out=w671:errorcluster)  [unwired: 2 in, 1 out]
              n216 = property on="历史波形图" class="WFGraph (strict)"(error in=w671, "Plot.Visible?"=w669) -> ()  [unwired: 1 in, 2 out]
            }
            n217 = property on="历史波形图" class="WFGraph (strict)"(error in=w659, "Cursor.Cursor Plot"=w652) -> (error out=w660:errorcluster)  [unwired: 1 in, 1 out]
            n218 = property on="历史波形图" class="WFGraph (strict)"(error in=w660, "Cursor.Cursor Plot"=w647) -> ()  [unwired: 1 in, 2 out]
            n219 = for {
              N: w653 -> [_]
              tunnel: w657 -> [w676] mode=indexing
              tunnel: "曲线标尺" -> [w674] mode=indexing
              shift-right: [w672] -> w654
              shift-left: bool[] [FALSE, FALSE, FALSE, FALSE, FALSE, FALSE, FALSE, FALSE] ("曲线标尺") -> [w677]
              n220 = Index Array(array=w677, index=w676) -> (element=w675:bool)
              n221 = Or(x=w674, y=w675) -> (x .or. y?=w673:bool)
              n222 = Replace Array Subset(array=w677, new element=w673, index=w676) -> (w672:bool[])
            }
            n223 = for {
              tunnel: w654 -> [w667] mode=indexing
              i -> [w668]
              n224 = property on="历史波形图" class="WFGraph (strict)"("ActYScl"=w668) -> (error out=w666:errorcluster)  [unwired: 2 in, 1 out]
              n225 = property on="历史波形图" class="WFGraph (strict)"(error in=w666, "YScale.Visible"=w667) -> ()  [unwired: 1 in, 2 out]
            }
          }
        }
        n226 = Subtract(x=w385, y=w401) -> (x-y=w452:i32)
        "临界段" <- w452
        n227 = Subtract(x=w396, y=w397) -> (x-y=w398:i32)
        "终端" <- w398
        n228 = Subtract(x=w397, y=w385) -> (x-y=w384:i32)
        "动态段" <- w384
        n229 = local write "提示信息"("循环计算中，请拖动游标以选择数据段！" ("提示信息")) -> ()
        n230 = Build Array(w401, w385) -> (w418:i32[])
        n231 = Array Subset(array=w381, index (col)=w397, length (col)=w398) -> (w395:dbl[][])  [unwired: 2 in]
        n232 = Array Subset(array=w386, index=w385, length=w384) -> (w393:dbl[])
        n233 = Array Subset(array=w458, index (col)=w401, length (col)=w452) -> (w457:dbl[][])  [unwired: 2 in]
        n234 = Array Subset(array=w381, index (col)=w401, length (col)=w452) -> (w453:dbl[][])  [unwired: 2 in]
        n235 = Array Subset(array=w381, index (col)=w385, length (col)=w384) -> (w402:dbl[][])  [unwired: 2 in]
        n236 = for {
          tunnel: w457 -> [w705] mode=indexing
          tunnel: w454 -> [w717]
          tunnel: w456 -> [w720]
          tunnel: w455 -> [w719]
          tunnel: w453 -> [w690] mode=indexing
          tunnel: [w692] -> w438 mode=indexing
          tunnel: [w689] -> w436 mode=indexing
          tunnel: [w718] -> w439 mode=indexing
          tunnel: [w696] -> w437 mode=indexing
          tunnel: w408 -> [w698]
          tunnel: T4 {"amp min"=-inf, "amp max"=inf, "damping min"=-inf, "damping max"=inf, "offset min"=0.0, "offset max"=0.0} ("parameter bounds") -> [w700]
          tunnel: w402 -> [w691] mode=indexing
          tunnel: w395 -> [w693] mode=indexing
          tunnel: w393 -> [w688]
          tunnel: "棒位偏移" -> [w687]
          tunnel: [w680] -> w377 mode=indexing
          tunnel: [w678] -> w379
          # "棒位"
          # "反应性"
          # "终端反应性数据"
          # "时间间隔"
          # "拟合周期"
          # "倒时方程计算反应性"
          n237 = Add(x=1.0, y=w687) -> (x+y=w685:dbl)
          n238 = Array Size(array=w705) -> (size(s)=w707:i32)
          n239 = for {
            N: w707 -> [_]
            tunnel: [w728] -> w706 mode=indexing
            i -> [w728]
          }
          n240 = Multiply(x=w688, y=w685) -> (x*y=w684:dbl[])
          n241 = Array Size(array=w684) -> (size(s)=w683:i32)
          n242 = Array Size(array=w690) -> (size(s)=w708:i32)
          n243 = call <vilib>:"Exponential Fit.vi"("Y"=w705, "X"=w706, "parameter bounds"=w700) -> ("damping"=w704:dbl)  [unwired: 7 in, 5 out]
          n244 = Less?(x=w683, y=1) -> (x < y?=w681:bool)
          n245 = Add Array Elements(numeric array=w690) -> (sum=w716:dbl)
          n246 = Divide(x=1.0, y=w704) -> (x/y=w699:dbl)
          n247 = Divide(x=w716, y=w708) -> (x/y=w689:dbl)
          n248 = Subtract(x=w691, y=w689) -> (x-y=w680:dbl[])
          n249 = Array Size(array=w680) -> (size(s)=w679:i32)
          n250 = case shown="True" w681 {
            tunnel: w684 -> [w721 _]
            tunnel: w679 -> [_ w724]
            tunnel: [w721 w722] -> w678
            frame False {
            }
            frame True {
              n251 = for {
                N: w724 -> [_]
                tunnel: w724 -> [w727]
                tunnel: [w725] -> w723 mode=indexing
                i -> [w726]
                n252 = Subtract(x=w727, y=w726) -> (x-y=w725:i32)
              }
              n253 = To Double Precision Float(number=w723) -> (double precision float=w722:dbl[])
            }
          }
          n254 = Multiply(x=w699, y=w698) -> (x*y=w697:dbl)
          n255 = Natural Logarithm(1:sgl 2.0) -> (0:w701:sgl)
          n256 = Array Size(array=w693) -> (size(s)=w694:i32)
          n257 = Multiply(x=w697, y=w701) -> (x*y=w696:dbl)
          n258 = Add Array Elements(numeric array=w693) -> (sum=w695:dbl)
          n259 = Divide(x=w695, y=w694) -> (x/y=w692:dbl)
          n260 = Multiply(x=w719, y=w697) -> (x*y=w709:dbl[])
          n261 = Increment(x=w709) -> (x+1=w710:dbl[])
          n262 = Divide(x=w717, y=w697) -> (x/y=w713:dbl)
          n263 = Divide(x=w720, y=w710) -> (x/y=w715:dbl[])
          n264 = Add Array Elements(numeric array=w715) -> (sum=w714:dbl)
          n265 = Add(x=w714, y=w713) -> (x+y=w712:dbl)
          n266 = Multiply(x=w712, y=sgl 100000.0) -> (x*y=w718:dbl)
        }
        "实时反应性 (pcm)" <- w436
        "终端反应性 (pcm)" <- w438
        "拟合反应性 (pcm)" <- w439
        "准临界周期 (s)" <- w437
        n267 = To Double Precision Float(number=w418) -> (double precision float=w417:dbl[])
        n268 = Insert Into Array(array=w377, index (row)=0 ("索引 (行)"), new element=w379) -> (w383:dbl[][])  [unwired: 1 in]
        n269 = Transpose 2D Array(2D array=w383) -> (transposed array=w382:dbl[][])
        n270 = for {
          N -> [w632]
          tunnel: w439 -> [w641] mode=indexing
          tunnel: w438 -> [w639] mode=indexing
          tunnel: w437 -> [w642] mode=indexing
          tunnel: w436 -> [w640] mode=indexing
          shift-right: [w636] -> w426
          shift-left: dbl[] [] -> [w638]
          shift-right: [w633] -> w429
          shift-left: string[] [] ("行首字符串[]") -> [w635]
          tunnel: [w632] -> w421
          n271 = Build Array(w642, w641, w640, w639) -> (w637:dbl[])
          n272 = Insert Into Array(array=w635, new element=string[] ["临界周期S", "拟合值PCM", "平均值PCM", "总价值PCM"] ("行首字符串[]")) -> (w633:string[])  [unwired: 1 in]
          n273 = Insert Into Array(array=w638, new element=w637) -> (w636:dbl[])  [unwired: 1 in]
        }
        n274 = Insert Into Array(array=w426, new element=w417) -> (w425:dbl[])  [unwired: 1 in]
        n275 = case shown="False" "添加记录" {
          tunnel: w434 -> [w607 w631]
          tunnel: w425 -> [_ w630]
          tunnel: [w606 w629] -> w424
          tunnel: [w605 TRUE] -> w432
          frame False {
            n276 = property on="Table" class="Tbl (strict)"() -> ("Selection Start"=w614:T6, "Selection Size"=w613:T6)  [unwired: 2 in, 2 out]
            n277 = Unbundle By Name(w614) -> ("Row"=w604:i32)
            n278 = Unbundle By Name(w613) -> ("Row"=w611:i32, "Column"=w601:i32)
            n279 = Equal?(x=1, y=w611) -> (x = y?=w603:bool)
            n280 = Greater Or Equal?(x=w601, y=4) -> (x >= y?=w602:bool)
            n281 = And(x=w603, y=w602) -> (x .and. y?=w609:bool)
            n282 = case shown="True" w609 {
              tunnel: "是否删除该行记录？" ("消息") -> [_ w622]
              tunnel: w604 -> [_ w620]
              tunnel: w607 -> [w616 w619]
              tunnel: [w616 w618] -> w606
              tunnel: [FALSE TRUE] -> w605
              frame False {
              }
              frame True {
                n283 = Two Button Dialog(message=w622) -> (T button?=w621:bool)  [unwired: 2 in]
                n284 = case shown="True" w621 {
                  tunnel: w620 -> [_ w627]
                  tunnel: w619 -> [w623 w626]
                  tunnel: [w623 w624] -> w618
                  frame False {
                  }
                  frame True {
                    n285 = Delete From Array(array=w626, length=1 ("长度"), index (row)=w627) -> (array with subset deleted=w624:dbl[][])  [unwired: 1 in, 1 out]
                  }
                }
              }
            }
          }
          frame True {
            n286 = Insert Into Array(array=w631, new element=w630) -> (w629:dbl[][])  [unwired: 2 in]
          }
        }
        n287 = Multiply(x=w421, y=4) -> (x*y=w419:i32)
        n288 = Array Size(array=w377) -> (size(s)=w373:i32[])
        n289 = Delete From Array(array=w424, length=2 ("长度"), index (col)=w419) -> (deleted portion=w416:dbl[][], array with subset deleted=w423:dbl[][])  [unwired: 1 in]
        n290 = Index Array(array=w373, index=0 ("索引")) -> (element=w369:i32)
        n291 = Array To Spreadsheet String(array=w382, 3:"%#g" ("格式字符串")) -> (spreadsheet string=w365:string)  [unwired: 1 in]
        n292 = local read "曲线隐显"() -> (w375:bool[])
        n293 = Array To Spreadsheet String(array=w423, 3:"%#g" ("格式字符串")) -> (spreadsheet string=w428:string)  [unwired: 1 in]
        n294 = case shown="True" "保存表格" {
          tunnel: w429 -> [_ w584]
          tunnel: w428 -> [_ w582]
          frame False {
          }
          frame True {
            n295 = Array To Spreadsheet String(array=w584, 3:"%s" ("格式字符串")) -> (spreadsheet string=w583:string)  [unwired: 1 in]
            n296 = File Dialog ("文件对话框")(6:"*.txt" ("类型（所有文件）"), 7:"请指定保存路径" ("提示"), 9:"总价值汇总.txt" ("默认名称")) -> (0:w575:errorcluster, 1:w576:bool, 3:w577:path)  [unwired: 1 in, 4 out]
            n297 = Concatenate Strings(w583, w582) -> (w581:string)
            n298 = case shown="False" w576 {
              tunnel: w581 -> [w587 _]
              tunnel: w577 -> [w586 _]
              frame False {
                n299 = Open/Create/Replace File(file path (use dialog)=w586, operation (0:open)=T5."replace or create") -> (refnum out=w590:refnum<file>, error out=w592:errorcluster)  [unwired: 4 in, 1 out]
                n300 = Write to Text File(file (use dialog)=w590, text=w587, error in=w592) -> (refnum out=w589:refnum<file>, error out=w588:errorcluster)  [unwired: 1 in, 1 out]
                n301 = Close File(refnum=w589, error in=w588) -> ()  [unwired: 2 out]
              }
              frame True {
              }
            }
            n302 = call <vilib>:"Clear Errors.vi"("error in (no error)"=w575) -> ()  [unwired: 5 in, 2 out]
          }
        }
        n303 = event shown="[0] \"Table\": Mouse Down" {
          selector: _ -> [_ _]
          dyn-events: _ -> [_ _]
          timeout: 20 -> [_ _]
          tunnel: w416 -> [w562 _]
          event "Table": Mouse Down {
            n304 = event-data() -> ("Mods"=w569:cluster{"Double Click":bool, "Menu Key":bool})  [unwired: 1 in]
            n305 = property on="Table" class="Tbl (strict)"() -> ("EditPos"=w567:T6)  [unwired: 2 in, 2 out]
            n306 = Unbundle By Name(w569) -> ("Double Click"=w565:bool)
            n307 = Unbundle By Name(w567) -> ("Row"=w561:i32)
            n308 = Greater Or Equal?(x=w561, y=0) -> (x >= y?=w566:bool)
            n309 = Index Array(array=w562, index (row)=w561) -> (element=w563:dbl[])  [unwired: 1 in]
            n310 = And(x=w565, y=w566) -> (x .and. y?=w564:bool)
            n311 = case shown="True" w564 {
              tunnel: w563 -> [_ w571]
              frame False {
              }
              frame True {
                n312 = To Long Integer(number=w571) -> (32bit integer=w570:i32[])
                n313 = for {
                  tunnel: w570 -> [w572] mode=indexing
                  i -> [w573]
                  n314 = property on="历史波形图" class="WFGraph (strict)"("Active Cursor"=w573) -> (error out=w574:errorcluster)  [unwired: 2 in, 1 out]
                  n315 = property on="历史波形图" class="WFGraph (strict)"(error in=w574, "Cursor.Cursor Index"=w572) -> ()  [unwired: 1 in, 2 out]
                }
              }
            }
          }
          event Timeout {
            n316 = event-data() -> ()  [unwired: 1 in, 1 out]
          }
        }
        n317 = Spreadsheet String To Array(format string="%s" ("格式字符串"), spreadsheet string=w365, array type (2D Dbl)=string[][] [] ("添加的数组")) -> (array=→"ValueTable":string[][])  [unwired: 1 in]
        n318 = for {
          N: w369 -> [_]
          tunnel: w375 -> [w503]
          shift-right: [w498] -> w371
          shift-left: bool[] [] -> [w497]
          i -> [w505]
          n319 = Multiply(x=2, y=w505) -> (x*y=w502:i32)
          n320 = Add(x=1, y=w502) -> (x+y=w500:i32)
          n321 = Index Array(array=w503, index=w500) -> (element=w499:bool)
          n322 = Insert Into Array(array=w497, new element=w499) -> (w498:bool[])  [unwired: 1 in]
        }
        n323 = for {
          N: w369 -> [_]
          tunnel: w376 -> [w494]
          shift-right: [w489] -> w366
          shift-left: string[] ["棒位"] ("添加的数组") -> [w488]
          i -> [w496]
          n324 = Multiply(x=2, y=w496) -> (x*y=w493:i32)
          n325 = Add(x=1, y=w493) -> (x+y=w491:i32)
          n326 = Index Array(array=w494, index=w491) -> (element=w490:string)
          n327 = Insert Into Array(array=w488, new element=w490) -> (w489:string[])  [unwired: 1 in]
        }
        n328 = case shown="True" w432 {
          tunnel: w429 -> [_ w594]
          tunnel: w428 -> [_ w593]
          frame False {
          }
          frame True {
            n329 = property on="Table" class="Tbl (strict)"("Column Headers[]"=w594, "Col Headers Vis"=TRUE ("显示项:显示列首")) -> (error out=w596:errorcluster)  [unwired: 2 in, 1 out]
            n330 = Spreadsheet String To Array(format string="%s" ("格式字符串"), spreadsheet string=w593, array type (2D Dbl)=string[][] [] ("添加的数组")) -> (array=→"Table":string[][])  [unwired: 1 in]
            n331 = property on="Table" class="Tbl (strict)"(error in=w596, "Selection Size"=T6 {"Row"=0, "Column"=0} ("选择区域大小")) -> ()  [unwired: 1 in, 2 out]
          }
        }
        n332 = for {
          tunnel: w379 -> [w506]
          tunnel: w377 -> [w507] mode=indexing
          tunnel: [w508] -> w378 mode=indexing
          n333 = Bundle "Bundle"(w506, w507) -> (w508:cluster{dbl[], dbl[]})  [unwired: 1 in]
        }
        "价值曲线" <- w378
        n334 = case shown="True" w368 {
          tunnel: w371 -> [_ w484]
          tunnel: w366 -> [_ w482]
          frame False {
          }
          frame True {
            n335 = for {
              tunnel: w484 -> [w486] mode=indexing
              i -> [w485]
              n336 = property on="价值曲线" class="XYGraph (strict)"("Active Plot"=w485) -> (error out=w487:errorcluster)  [unwired: 2 in, 1 out]
              n337 = property on="价值曲线" class="XYGraph (strict)"(error in=w487, "Plot.Visible?"=w486) -> ()  [unwired: 1 in, 2 out]
            }
            n338 = property on="ValueTable" class="Tbl (strict)"("Column Headers[]"=w482, "Col Headers Vis"=TRUE ("显示项:显示列首")) -> ()  [unwired: 2 in, 2 out]
          }
        }
        n339 = local read "退出程序"() -> (w450:bool)
        n340 = case shown="True" "另存数据" {
          tunnel: w366 -> [_ w473]
          tunnel: w365 -> [_ w471]
          frame False {
          }
          frame True {
            n341 = Array To Spreadsheet String(array=w473, 3:"%s" ("格式字符串")) -> (spreadsheet string=w472:string)  [unwired: 1 in]
            n342 = File Dialog ("文件对话框")(6:"*.txt" ("类型（所有文件）"), 7:"请指定保存路径" ("提示"), 9:"棒价值数据.txt" ("默认名称")) -> (0:w464:errorcluster, 1:w465:bool, 3:w466:path)  [unwired: 1 in, 4 out]
            n343 = Concatenate Strings(w472, w471) -> (w470:string)
            n344 = case shown="False" w465 {
              tunnel: w470 -> [w476 _]
              tunnel: w466 -> [w475 _]
              frame False {
                n345 = Open/Create/Replace File(file path (use dialog)=w475, operation (0:open)=T5."replace or create") -> (refnum out=w479:refnum<file>, error out=w481:errorcluster)  [unwired: 4 in, 1 out]
                n346 = Write to Text File(file (use dialog)=w479, text=w476, error in=w481) -> (refnum out=w478:refnum<file>, error out=w477:errorcluster)  [unwired: 1 in, 1 out]
                n347 = Close File(refnum=w478, error in=w477) -> ()  [unwired: 2 out]
              }
              frame True {
              }
            }
            n348 = call <vilib>:"Clear Errors.vi"("error in (no error)"=w464) -> ()  [unwired: 5 in, 2 out]
          }
        }
      }
    }
    frame #3 {
      n349 = invoke class="VI" method="FP.Close"() -> (reference out=w730:refnum<vi>, error out=w729:errorcluster)  [unwired: 3 in, 1 out]
      n350 = Close Reference(reference=w730, error in (no error)=w729) -> ()  [unwired: 1 out]
    }
  }
  n351 = property class="Clust (strict)"("Visible"=w1) -> ()  [unwired: 2 in, 2 out]
  n352 = property on="刻棒选择" class="Ring (strict)"("Visible"=w1) -> ()  [unwired: 2 in, 2 out]
